vi "sub_vi_abs_rel_errors.vi"(2 "Measure":dbl, 3 "Min":dbl, 4 "Max":dbl) -> (0 "Relative error":dbl, 1 "Absolute error":dbl)   [LabVIEW 2016]
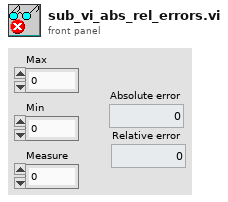
[diagram p1: front panel]
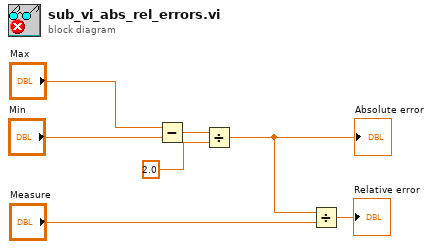
[diagram p0: block diagram]
diagram:
  n1 = Subtract(x="Max", y="Min") -> (x-y=w7:dbl)
  n2 = Divide(x=w7, y=2.0) -> (x/y=w5:dbl)
  "Absolute error" <- w5
  n3 = Divide(x=w5, y="Measure") -> (x/y=→"Relative error":dbl)
